vi "Homework 1.vi"() -> ()   [LabVIEW 2018]
doc: "CSC 470I Intro to Robotics, Homework/Module 1"
panel:
  out "Minutes":dbl(knob) scale=0.0..60.0
  out "Second(s)":i32(knob) scale=0.0..60.0
  out "Second(s)":dbl
  out "Minute(s)":dbl
  in  "stop":bool
  out "X ^ Y:":dbl
  out "Division:":dbl
  out "Multiplication:":dbl
  out "Subtraction:":dbl
  out "Addition:":dbl
  in  "Input #2":dbl
  in  "Input #1":dbl
  # "Results"
  # "Calculation Values"
  # "Time Elapsed"
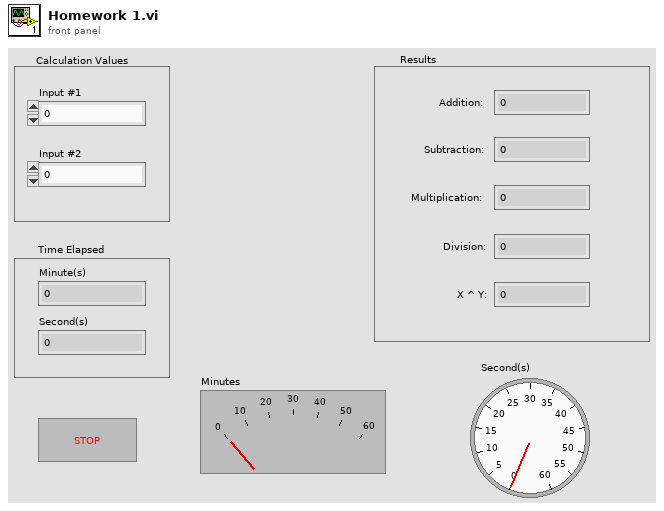
[diagram p1: front panel]
types:
  T1 = typedef "LVDateTimeRec.ctl" = cluster{"fractional second":dbl, "second":i32, "minute":i32, "hour":i32, "day of month":i32, "month":i32, "year":i32, "day of week":i32, "day of year":i32, "DST":i32}
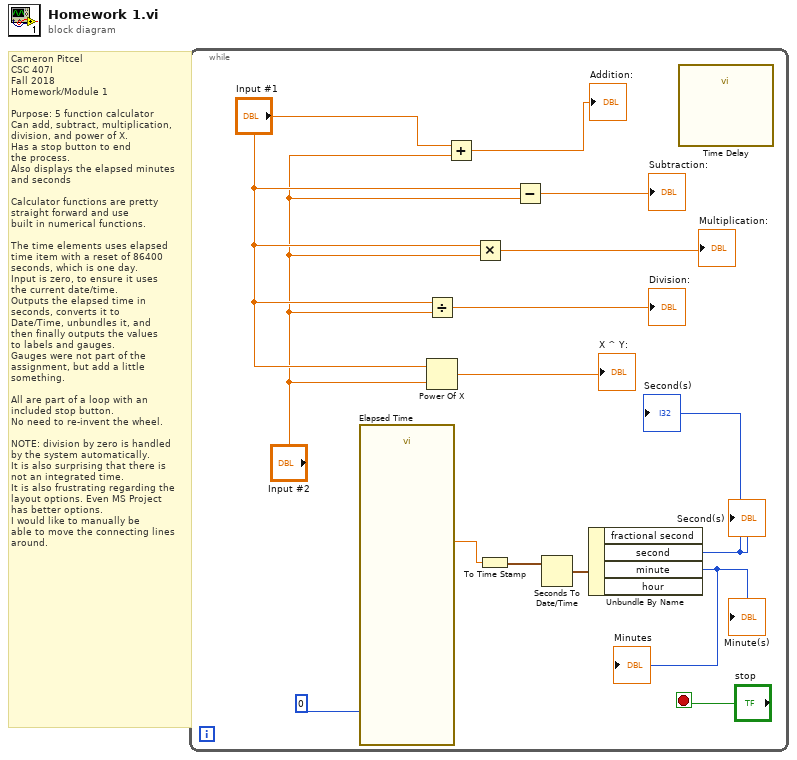
[diagram p0: block diagram]
diagram:
  # "Cameron Pitcel\nCSC 407I\nFall 2018\nHomework/Module 1\n\nPurpose: 5 function calculator\nCan add, subtract, multiplication,\ndivision, and power of X.\nHas a stop button to end\nthe process.\nAlso displays the elapsed minutes\nand seconds\n\nCalculator functions are pretty\nstraight forward and use \nbuilt in numerical functions.\n\nThe time elements uses elapsed \ntime item with a reset of 86400\nseconds, which is one day.\nInput is zero, to ensure it uses\nthe current date/time.\nOutputs the elapsed time in \nseconds, converts it to \nDate/Time, unbundles it, and\nthen finally outputs the values\nto labels and gauges.\nGauges were not part of the\nassignment, but add a little\nsomething.\n\nAll are part of a loop with an \nincluded stop button.\nNo need to re-invent the wheel.\n\nNOTE: division by zero is handled\nby the system automatically.\nIt is also surprising that there is\nnot an integrated time.\nIt is also frustrating regarding the\nlayout options. Even MS Project\nhas better options.\nI would like to manually be\nable to move the connecting lines\naround."
  n1 = while {
    stop <- "stop" stop-if-true
    n2 = call "Elapsed Time"("Set Start Time (s)"=0) -> ("Elapsed Time (s)"=w3:dbl)  [unwired: 11 in, 7 out]
    n3 = Divide(x="Input #1", y="Input #2") -> (x/y=→"Division:":dbl)
    n4 = Power Of X(1:"Input #2", 2:"Input #1") -> (0:→"X ^ Y:":dbl)
    n5 = Add(x="Input #1", y="Input #2") -> (x+y=→"Addition:":dbl)
    n6 = Multiply(x="Input #1", y="Input #2") -> (x*y=→"Multiplication:":dbl)
    n7 = To Time Stamp(1:w3) -> (0:w5:timestamp)
    n8 = Subtract(x="Input #1", y="Input #2") -> (x-y=→"Subtraction:":dbl)
    n9 = Seconds To Date/Time(time stamp (now)=w5) -> (date time rec=w4:T1)  [unwired: 1 in]
    n10 = Unbundle By Name(w4) -> ("second"=→"Second(s)" →"Second(s)":i32, "minute"=→"Minute(s)" →"Minutes":i32)  [unwired: 2 out]
    n11 = call "Time Delay"() -> ()  [unwired: 11 in, 1 out]
  }
